vi "Final 3.vi"(0 "Image In":T1, 7 "error in":errorcluster) -> (20 "Image Out":T1, 21 "String (OCR/OCV 1)":string, 22 "Classifier Session (Color Classification 1)":T2, 23 "Classes (Color Classification 1)":string[](array[string]), 24 "Number of Matches (Color Location 1)":i32, 25 "Number of Matches (Color Location 2)":i32, 27 "error out":errorcluster)   [LabVIEW 2019]
uses:
  <vilib>/vision/Image Controls.llb/IMAQ Image.ctl
  <vilib>/vision/Classification.llb/IMAQ Classifier Session.ctl
  <vilib>/vision/Classification.llb/IMAQ Classifier Read Options.ctl
  <vilib>/vision/NI_Vision_Development_Module.lvlib
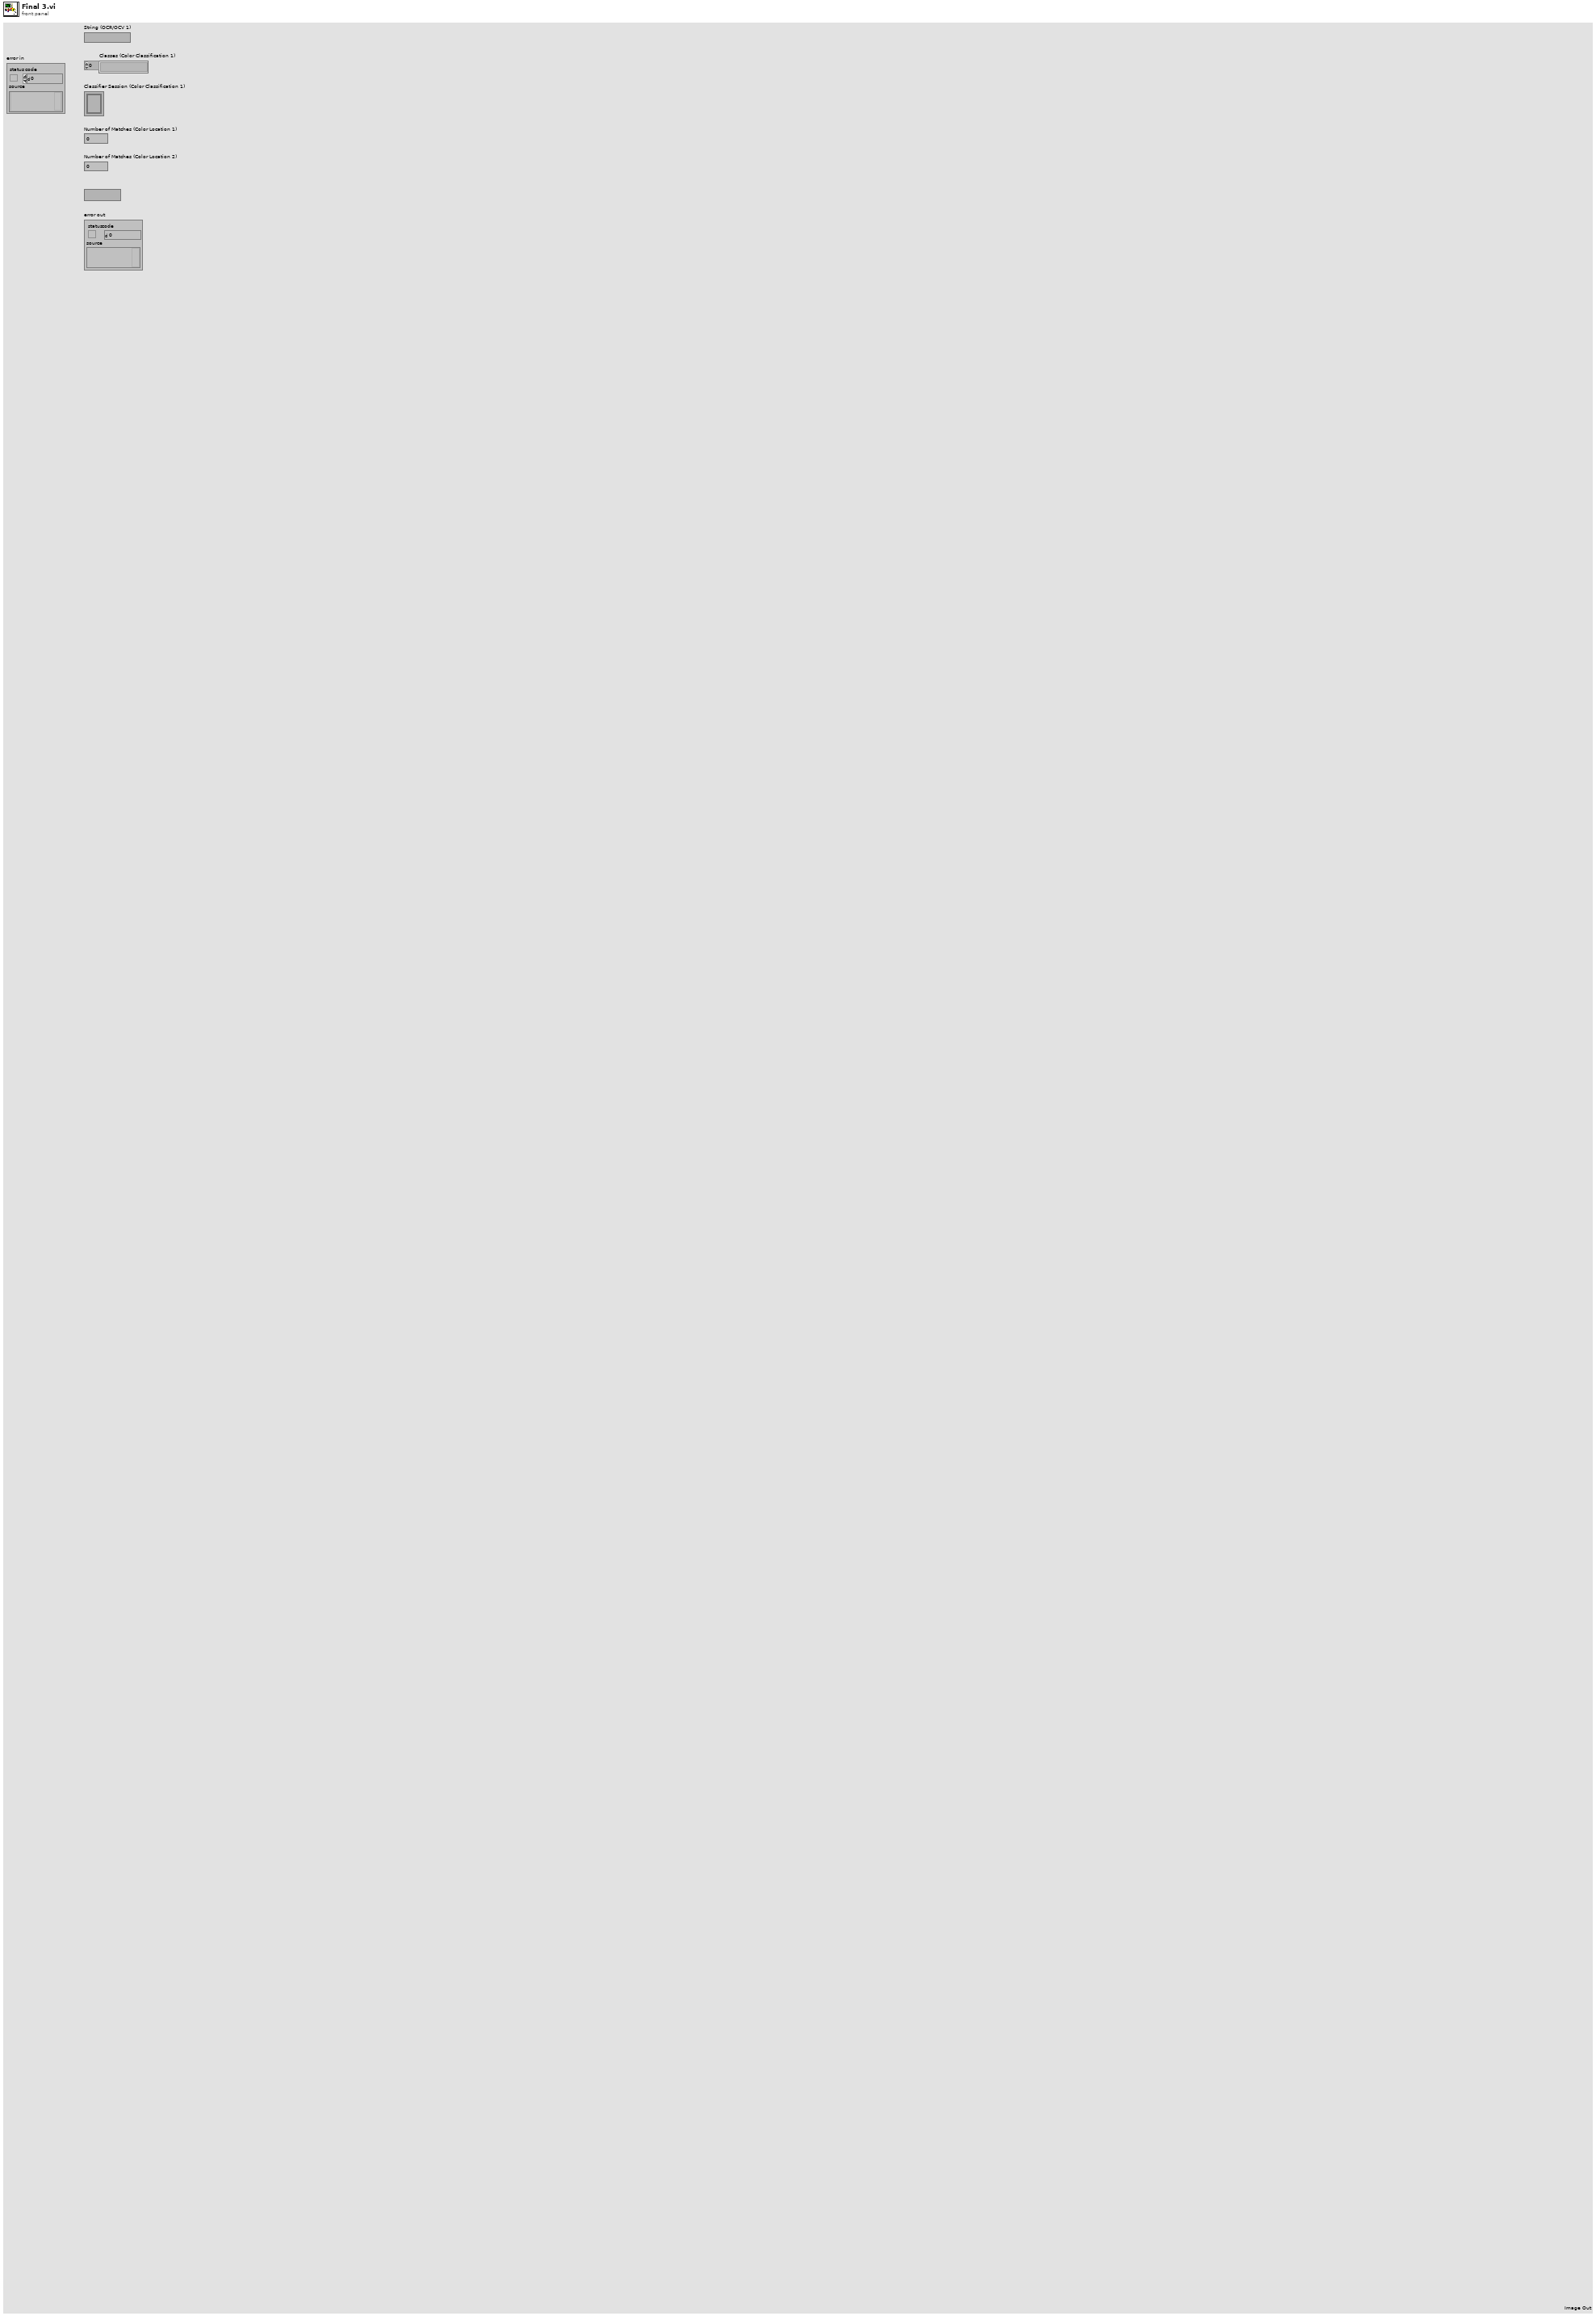
[diagram p1: front panel]
types:
  T1 = typedef "IMAQ Image.ctl" = refnum<image>
  T2 = typedef "IMAQ Classifier Session.ctl" = refnum<k1>
  T3 = typedef "Image Type" = u32
  T4 = cluster{"Global Rectangle":i32[], "Contours":cluster{"ID":enum32{"External", "Internal"}, "Type":u32, "Coordinates":i32[]}[]}
  T5 = cluster{"Threshold Data":cluster{"Method":enum16{"Fixed Range", "Uniform", "Linear", "Non Linear", "Local", "Color"}, "Looking for":u32, "Color Mode":u32, "Kernel Size":cluster{"Width":i32, "Height":i32}, "Ranges":cluster{"Min":i32, "Max":i32}[]}, "Reject Border":bool, "Number Of Erosions":i32, "Size & Spacing":cluster{"Segment Algorithm":u16, "Min Bounding Rect Width":i32, "Max Bounding Rect Width":i32, "Min Bounding Rect Height":i32, "Max Bounding Rect Height":i32, "Min Character Size":i32, "Max Character Size":i32, "Min Char Spacing":i32, "Max Horiz Element Spacing":i32, "Max Vert Element Spacing":i32, "Max Space Distance":i32}, "Read Options":cluster{"Read Strategy":i32, "Read Resolution":i32, "Scale Dependant":bool, "Aspect Ratio":i32, "Acceptance Level":i32, "Substitution Character":string, "MultiLine":bool}, "Valid Characters":cluster{"Pre-defined characters":i32, "User-defined characters":string}[], "Use Text Pattern":bool, "Orientation":u32, "# Lines Expected":u32, "Number of Blocks":i32}
  T6 = typedef "IMAQ OCR Session.ctl" = refnum<k1>
  T7 = typedef "IMAQ Classifier Read Options.ctl" = i32
  T8 = typedef "ROI Descriptor" = cluster{"Global Rectangle":i32[], "Contours":cluster{"ID":enum32{"External", "Internal"}, "Type":u32, "Coordinates":i32[]}[]}
  T9 = cluster{"Position":cluster{"x":sgl, "y":sgl}, "Angle":sgl, "Scale":sgl, "Score":sgl, "Bounding Box":cluster{"x":sgl, "y":sgl}[]}[]
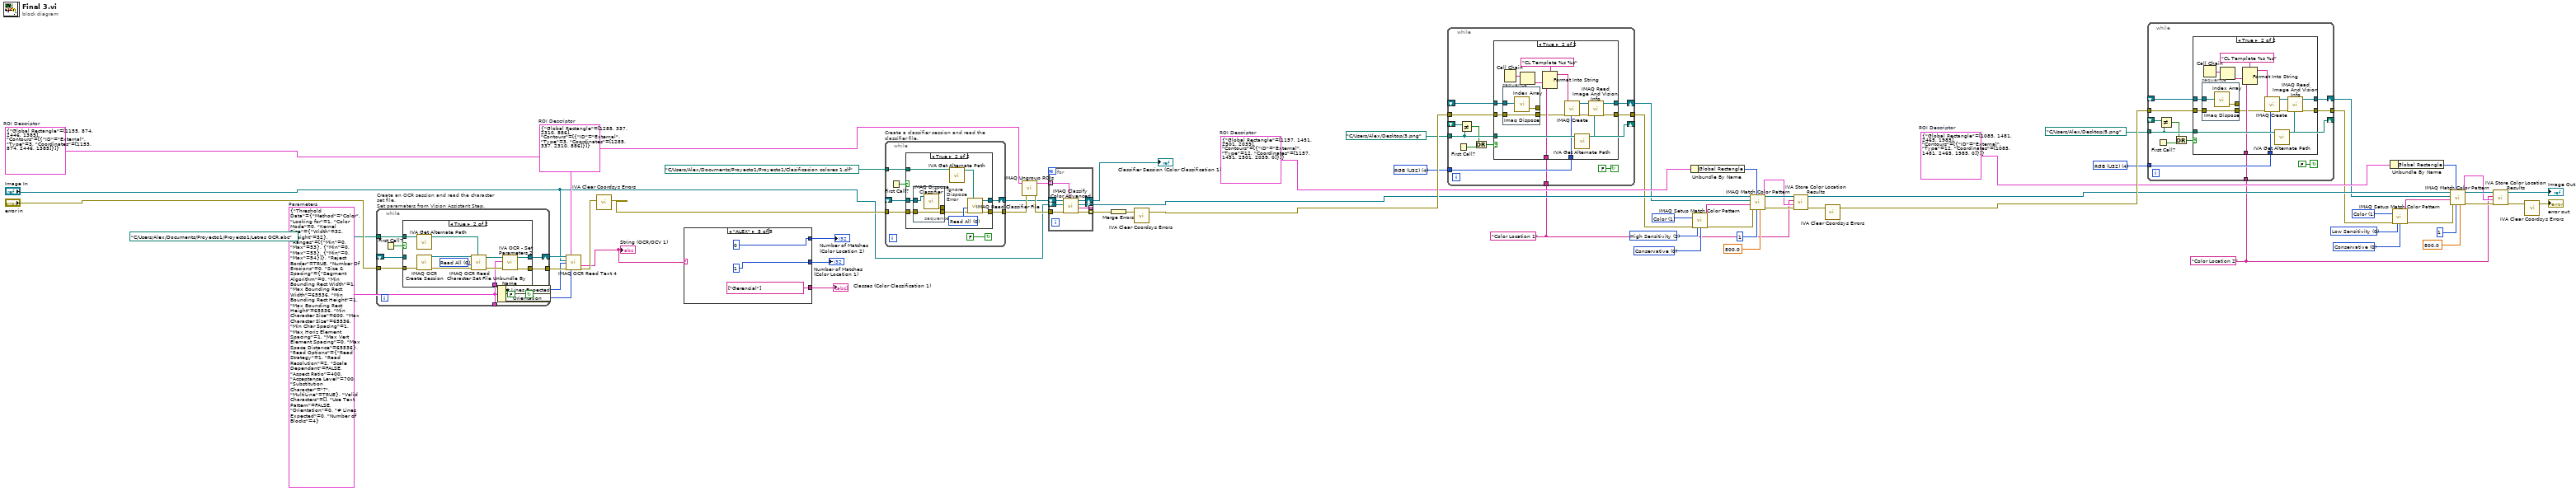
[diagram p0: block diagram]
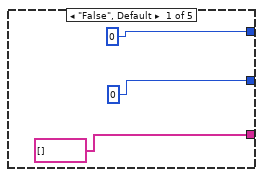
[diagram p2: hidden frame]
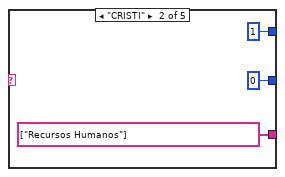
[diagram p3: hidden frame]
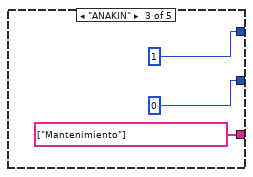
[diagram p4: hidden frame]
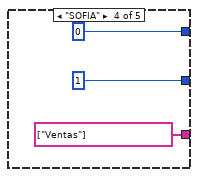
[diagram p5: hidden frame]
diagram:
  w12 = "Color Location 2" ("Step Name")
  w18 = T3 4 items=["Grayscale (U8)", "Grayscale (I16)", "Grayscale (SGL)", "Complex (CSG)", "RGB (U32)", "HSL (U32)", "RGB (U64)"] ("Image Type")
  w20 = u32 0 items=["Conservative", "Balance", "Aggressive", "Very Aggressive"] ("Search Strategy")
  w21 = u32 0 items=["Low Sensitivity", "Medium Sensitivity", "High Sensitivity"] ("Color Sensitivity")
  w22 = u32 1 items=["Color and Shape", "Color", "Shape"] ("Match Feature Mode")
  w17 = T4 {"Global Rectangle"=[1085, 1481, 2465, 1985], "Contours"=[{"ID"=enum."External", "Type"=12, "Coordinates"=[1085, 1481, 2465, 1985, 0]}]}  # ROI Descriptor
  w32 = "Color Location 1" ("Step Name")
  w37 = T3 4 items=["Grayscale (U8)", "Grayscale (I16)", "Grayscale (SGL)", "Complex (CSG)", "RGB (U32)", "HSL (U32)", "RGB (U64)"] ("Image Type")
  w39 = u32 0 items=["Conservative", "Balance", "Aggressive", "Very Aggressive"] ("Search Strategy")
  w40 = u32 2 items=["Low Sensitivity", "Medium Sensitivity", "High Sensitivity"] ("Color Sensitivity")
  w41 = u32 1 items=["Color and Shape", "Color", "Shape"] ("Match Feature Mode")
  w36 = T4 {"Global Rectangle"=[1157, 1451, 2501, 2039], "Contours"=[{"ID"=enum."External", "Type"=12, "Coordinates"=[1157, 1451, 2501, 2039, 0]}]}  # ROI Descriptor
  w53 = T4 {"Global Rectangle"=[1285, 337, 2310, 886], "Contours"=[{"ID"=enum."External", "Type"=3, "Coordinates"=[1285, 337, 2310, 886]}]}  # ROI Descriptor
  w61 = T5 {"Threshold Data"={"Method"=enum."Color", "Looking for"=1, "Color Mode"=0, "Kernel Size"={"Width"=32, "Height"=32}, "Ranges"=[{"Min"=0, "Max"=53}, {"Min"=0, "Max"=53}, {"Min"=0, "Max"=54}]}, "Reject Border"=TRUE, "Number Of Erosions"=0, "Size & Spacing"={"Segment Algorithm"=0, "Min Bounding Rect Width"=1, "Max Bounding Rect Width"=65536, "Min Bounding Rect Height"=1, "Max Bounding Rect Height"=65536, "Min Character Size"=600, "Max Character Size"=65536, "Min Char Spacing"=1, "Max Horiz Element Spacing"=1, "Max Vert Element Spacing"=0, "Max Space Distance"=65536}, "Read Options"={"Read Strategy"=1, "Read Resolution"=2, "Scale Dependant"=FALSE, "Aspect Ratio"=400, "Acceptance Level"=700, "Substitution Character"="?", "MultiLine"=TRUE}, "Valid Characters"=[], "Use Text Pattern"=FALSE, "Orientation"=0, "# Lines Expected"=0, "Number of Blocks"=4}  # Parameters
  w62 = T4 {"Global Rectangle"=[1155, 874, 2446, 1385], "Contours"=[{"ID"=enum."External", "Type"=3, "Coordinates"=[1155, 874, 2446, 1385]}]}  # ROI Descriptor
  n1 = while "Create an OCR session and read the character set file.\nSet paramaters from Vision Assistant Step." {
    shift-right: [w69] -> w59
    shift-left: _ -> [w68]
    tunnel: "error in" -> [w71]
    tunnel: w61 -> [w67]
    tunnel: path "C:/Users/Alex/Documents/Proyecto1/Proyecto1/Letras OCR.abc" ("File Path") -> [w66]
    tunnel: [w65] -> w60
    stop <- FALSE continue-if-true
    n2 = First Call?() -> (First Call?: T/F=w70:bool)
    n3 = case shown="True" w70 {
      tunnel: w66 -> [_ w78]
      tunnel: w71 -> [w73 w82]
      tunnel: [w74 w80] -> w69
      tunnel: [w73 w79] -> w65
      tunnel: w67 -> [_ w75]
      tunnel: w68 -> [w74 _]
      frame False {
      }
      frame True {
        w83 = 0 items=["Read All", "Read Character Set Only", "Read Properties Only"] ("Read Options")
        n4 = call <vilib>:"IVA Get Alternate Path.vi"("Path In"=w78) -> ("Path Out"=w77:path)  [unwired: 10 out]
        n5 = call "IMAQ OCR Create Session"("error in (no error)"=w82) -> ("error out"=w84:errorcluster, "IMAQ OCR Session"=w85:T6)  [unwired: 9 out]
        n6 = call "IMAQ OCR Read Character Set File"("File Path"=w77, "error in (no error)"=w84, "Read Options"=w83, "IMAQ OCR Session"=w85) -> ("error out"=w81:errorcluster, "IMAQ OCR Session (dup)"=w76:T6)  [unwired: 1 in, 5 out]
        n7 = call <vilib>:"IVA OCR - Set Parameters 2.vi"("error in (no error)"=w81, "Parameters"=w75, "IMAQ OCR Session"=w76) -> ("error out"=w79:errorcluster, "IMAQ OCR Session Out"=w80:T6)  [unwired: 7 in]
      }
    }
  }
  n8 = Unbundle By Name(w61) -> ("# Lines Expected"=w57:u32, "Orientation"=w58:u32)
  n9 = call "IMAQ OCR Read Text 4"("IMAQ OCR Session"=w59, "ROI Descriptor"=w62, "Image"="Image In", "Number of Lines Requested"=w57, "error in (no error)"=w60, "Orientation"=w58) -> ("Read String"=w4:string, "error out"=w56:errorcluster)  [unwired: 8 out]
  "String (OCR/OCV 1)" <- w4
  n10 = call <vilib>:"IVA Clear Coordsys Errors.vi"("error in (no error)"=w56) -> ("error out"=w55:errorcluster)  [unwired: 10 in]
  n11 = case shown="\"ALEX\"" w4 {
    tunnel: [0 ("Number of Matches (Color Location 2)") 1 ("Number of Matches (Color Location 2)") 1 ("Number of Matches (Color Location 2)") 0 ("Number of Matches (Color Location 2)") 0 ("Number of Matches (Color Location 2)")] -> w3
    tunnel: [0 ("Number of Matches (Color Location 1)") 0 ("Number of Matches (Color Location 1)") 0 ("Number of Matches (Color Location 1)") 1 ("Number of Matches (Color Location 1)") 1 ("Number of Matches (Color Location 1)")] -> w2
    tunnel: [string[] [] ("Classes (Color Classification 1)") string[] ["Recursos Humanos"] ("Classes (Color Classification 1)") string[] ["Mantenimiento"] ("Classes (Color Classification 1)") string[] ["Ventas"] ("Classes (Color Classification 1)") string[] ["Gerencial"] ("Classes (Color Classification 1)")] -> w1
    frame "False", Default {
    }
    frame "CRISTI" {
    }
    frame "ANAKIN" {
    }
    frame "SOFIA" {
    }
    frame "ALEX" {
    }
  }
  "Classes (Color Classification 1)" <- w1
  "Number of Matches (Color Location 1)" <- w2
  "Number of Matches (Color Location 2)" <- w3
  n12 = while "Create a classifier session and read the classifier file." {
    shift-right: [w107] -> w45
    shift-left: _ -> [w106]
    tunnel: w55 -> [w104]
    tunnel: [w103] -> w52
    tunnel: path "C:/Users/Alex/Documents/Proyecto1/Proyecto1/Clasificacion colores 1.clf" ("File Path") -> [w102]
    stop <- FALSE continue-if-true
    n13 = First Call?() -> (First Call?: T/F=w101:bool)
    n14 = case shown="True" w101 {
      tunnel: [w109 w116] -> w107
      tunnel: w106 -> [w109 w114]
      tunnel: w104 -> [w108 w113]
      tunnel: [w108 w115] -> w103
      tunnel: w102 -> [_ w111]
      frame False {
      }
      frame True {
        w117 = T7 0 items=["Read All", "Add Samples, Do Not Change Options", "Read Options, Do Not Add Samples"] ("Read Options")
        # "Ignore Dispose Error"
        n15 = stacked-sequence {
          tunnel: w114 -> [w120]
          tunnel: w113 -> [w119]
          tunnel: [w119] -> w112
          tunnel: [w118] -> _
          frame #0 {
            n16 = call "IMAQ Dispose Classifier"("Classifier Session"=w120) -> ("error out"=w118:errorcluster)  [unwired: 1 in, 9 out]
          }
        }
        n17 = call <vilib>:"IVA Get Alternate Path.vi"("Path In"=w111) -> ("Path Out"=w110:path)  [unwired: 10 out]
        n18 = call "IMAQ Read Classifier File"("File Path"=w110, "error in (no error)"=w112, "Read Options"=w117) -> ("error out"=w115:errorcluster, "Classifier Session"=w116:T2)  [unwired: 1 in, 6 out]
      }
    }
  }
  n19 = call "IMAQ Ungroup ROIs"("error in (no error)"=w52, "ROI Descriptor"=w53) -> ("error out"=w51:errorcluster, "ROI Descriptors out"=w50:T8[])  [unwired: 2 out]
  n20 = for {
    tunnel: [w128] -> _ mode=indexing
    tunnel: [w127] -> w49 mode=indexing
    tunnel: w51 -> [w125]
    tunnel: w50 -> [w124] mode=indexing
    shift-right: [w122] -> w34
    shift-left: "Image In" -> [w123]
    shift-right: [w121] -> w44
    shift-left: w45 -> [w126]
    n21 = call "IMAQ Classify Color Advanced"("ROI Descriptor"=w124, "error in (no error)"=w125, "Image"=w123, "Classifier Session"=w126) -> ("error out"=w127:errorcluster, "Class"=w128:string, "Image (dup)"=w122:T1, "Classifier Session (dup)"=w121:T2)  [unwired: 4 out]
  }
  "Classifier Session (Color Classification 1)" <- w44
  n22 = Merge Errors(w49) -> (w48:errorcluster)
  n23 = call <vilib>:"IVA Clear Coordsys Errors.vi"("error in (no error)"=w48) -> ("error out"=w47:errorcluster)  [unwired: 10 in]
  n24 = while {
    shift-right: [w140] -> w28
    shift-left: _ -> [w139]
    tunnel: [w137] -> w27
    tunnel: w47 -> [w136]
    tunnel: path "C:/Users/Alex/Desktop/3.png" ("File Path") -> [w132]
    tunnel: w37 -> [w135]
    tunnel: w32 -> [w134]
    shift-right: [w132] -> _
    shift-left: _ -> [w133]
    stop <- FALSE continue-if-true
    n25 = First Call?() -> (First Call?: T/F=w131:bool)
    n26 = Not Equal?(x=w133, y=w132) -> (x != y?=w130:bool)
    n27 = Or(x=w130, y=w131) -> (x .or. y?=w129:bool)
    n28 = case shown="True" w129 {
      tunnel: [w142 w155] -> w140
      tunnel: w139 -> [w142 w147]
      tunnel: [w141 w152] -> w137
      tunnel: w136 -> [w141 w146]
      tunnel: w135 -> [_ w151]
      tunnel: w134 -> [_ w148]
      tunnel: w132 -> [_ w144]
      frame False {
      }
      frame True {
        n29 = Call Chain() -> (call chain=w150:string[])
        n30 = stacked-sequence {
          tunnel: w147 -> [w160]
          tunnel: w146 -> [w159]
          tunnel: [w159] -> w145
          tunnel: [w158] -> _
          frame #0 {
            n31 = call "Imaq Dispose"("Image"=w160) -> ("error out"=w158:errorcluster)  [unwired: 2 in, 3 out]
          }
        }
        n32 = Index Array(array=w150) -> (element=w149:string)  [unwired: 1 in]
        n33 = Format Into String(format string="CL Template %s %s" ("Image Name"), w149, w148) -> (resulting string=w157:string)  [unwired: 2 in, 1 out]
        n34 = call "IMAQ Create"("Image Name"=w157, "Image Type"=w151, "error in (no error)"=w145) -> ("New Image"=w154:T1, "error out"=w153:errorcluster)  [unwired: 1 in, 1 out]
        n35 = call <vilib>:"IVA Get Alternate Path.vi"("Path In"=w144) -> ("Path Out"=w143:path)  [unwired: 10 out]
        n36 = call "IMAQ Read Image And Vision Info"("File Path"=w143, "error in (no error)"=w153, "Image"=w154) -> ("error out"=w152:errorcluster, "Image Out"=w155:T1)  [unwired: 1 in, 6 out]
      }
    }
  }
  n37 = Unbundle By Name(w36) -> ("Global Rectangle"=w29:i32[])
  n38 = call "IMAQ Setup Match Color Pattern"("Match Feature Mode"=w41, "error in (no error)"=w27, "Color Sensitivity"=w40, "Search Strategy"=w39) -> ("Match Color Pattern Setup Data"=w31:string, "error out"=w30:errorcluster)  [unwired: 5 in, 5 out]
  n39 = call "IMAQ Match Color Pattern"("Minimum Match Score"=sgl 800.0, "Number of Matches Requested"=1, "Optional Rectangle"=w29, "error in (no error)"=w30, "Match Color Pattern Setup Data"=w31, "Template Image"=w28, "Image"=w34) -> ("error out"=w35:errorcluster, "Matches"=w33:T9)  [unwired: 3 out]
  n40 = call <vilib>:"IVA Store Color Location Results.vi"("error in (no error)"=w35, "Matches"=w33, "Step Name"=w32, "Image in"=w34) -> ("error out"=w26:errorcluster, "Image dup"=w14:T1)  [unwired: 6 out]
  n41 = call <vilib>:"IVA Clear Coordsys Errors.vi"("error in (no error)"=w26) -> ("error out"=w25:errorcluster)  [unwired: 10 in]
  n42 = while {
    shift-right: [w172] -> w8
    shift-left: _ -> [w171]
    tunnel: [w169] -> w7
    tunnel: w25 -> [w168]
    tunnel: path "C:/Users/Alex/Desktop/5.png" ("File Path") -> [w164]
    tunnel: w18 -> [w167]
    tunnel: w12 -> [w166]
    shift-right: [w164] -> _
    shift-left: _ -> [w165]
    stop <- FALSE continue-if-true
    n43 = First Call?() -> (First Call?: T/F=w163:bool)
    n44 = Not Equal?(x=w165, y=w164) -> (x != y?=w162:bool)
    n45 = Or(x=w162, y=w163) -> (x .or. y?=w161:bool)
    n46 = case shown="True" w161 {
      tunnel: [w174 w187] -> w172
      tunnel: w171 -> [w174 w179]
      tunnel: [w173 w184] -> w169
      tunnel: w168 -> [w173 w178]
      tunnel: w167 -> [_ w183]
      tunnel: w166 -> [_ w180]
      tunnel: w164 -> [_ w176]
      frame False {
      }
      frame True {
        n47 = Call Chain() -> (call chain=w182:string[])
        n48 = stacked-sequence {
          tunnel: w179 -> [w192]
          tunnel: w178 -> [w191]
          tunnel: [w191] -> w177
          tunnel: [w190] -> _
          frame #0 {
            n49 = call "Imaq Dispose"("Image"=w192) -> ("error out"=w190:errorcluster)  [unwired: 2 in, 3 out]
          }
        }
        n50 = Index Array(array=w182) -> (element=w181:string)  [unwired: 1 in]
        n51 = Format Into String(format string="CL Template %s %s" ("Image Name"), w181, w180) -> (resulting string=w189:string)  [unwired: 2 in, 1 out]
        n52 = call "IMAQ Create"("Image Name"=w189, "Image Type"=w183, "error in (no error)"=w177) -> ("New Image"=w186:T1, "error out"=w185:errorcluster)  [unwired: 1 in, 1 out]
        n53 = call <vilib>:"IVA Get Alternate Path.vi"("Path In"=w176) -> ("Path Out"=w175:path)  [unwired: 10 out]
        n54 = call "IMAQ Read Image And Vision Info"("File Path"=w175, "error in (no error)"=w185, "Image"=w186) -> ("error out"=w184:errorcluster, "Image Out"=w187:T1)  [unwired: 1 in, 6 out]
      }
    }
  }
  n55 = Unbundle By Name(w17) -> ("Global Rectangle"=w9:i32[])
  n56 = call "IMAQ Setup Match Color Pattern"("Match Feature Mode"=w22, "error in (no error)"=w7, "Color Sensitivity"=w21, "Search Strategy"=w20) -> ("Match Color Pattern Setup Data"=w11:string, "error out"=w10:errorcluster)  [unwired: 5 in, 5 out]
  n57 = call "IMAQ Match Color Pattern"("Minimum Match Score"=sgl 800.0, "Number of Matches Requested"=1, "Optional Rectangle"=w9, "error in (no error)"=w10, "Match Color Pattern Setup Data"=w11, "Template Image"=w8, "Image"=w14) -> ("error out"=w16:errorcluster, "Matches"=w13:T9)  [unwired: 3 out]
  n58 = call <vilib>:"IVA Store Color Location Results.vi"("error in (no error)"=w16, "Matches"=w13, "Step Name"=w12, "Image in"=w14) -> ("error out"=w6:errorcluster, "Image dup"=→"Image Out":T1)  [unwired: 6 out]
  n59 = call <vilib>:"IVA Clear Coordsys Errors.vi"("error in (no error)"=w6) -> ("error out"=→"error out":errorcluster)  [unwired: 10 in]
